vi "TCP Write.vi"(3 "error in (no error)":errorcluster, 4 "Data to Write":T1={"Array of Motor Speeds"=[0.0, 0.0, 0.0, 0.0]}, 5 "connection ID":refnum<k5>) -> (0 "error out":errorcluster, 2 "connection ID out":refnum<k5>)   [LabVIEW 2018]
uses:
  controls/TCP Write select.ctl
panel:
  # "Use this code as a starting point. This VI should take the values from the cluster\nand write them all on TCP."
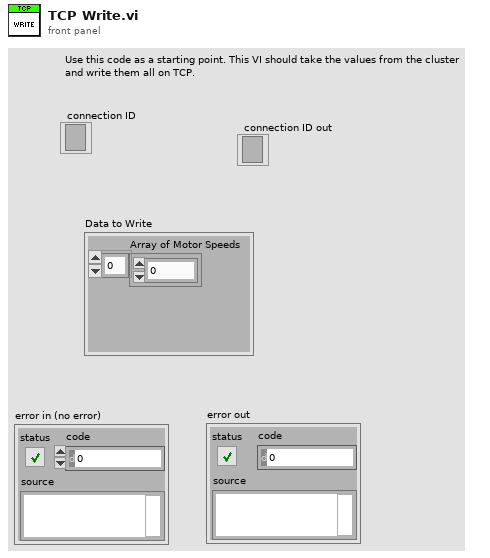
[diagram p1: front panel]
types:
  T1 = typedef "TCP Write select.ctl" = cluster{"Array of Motor Speeds":dbl[]}
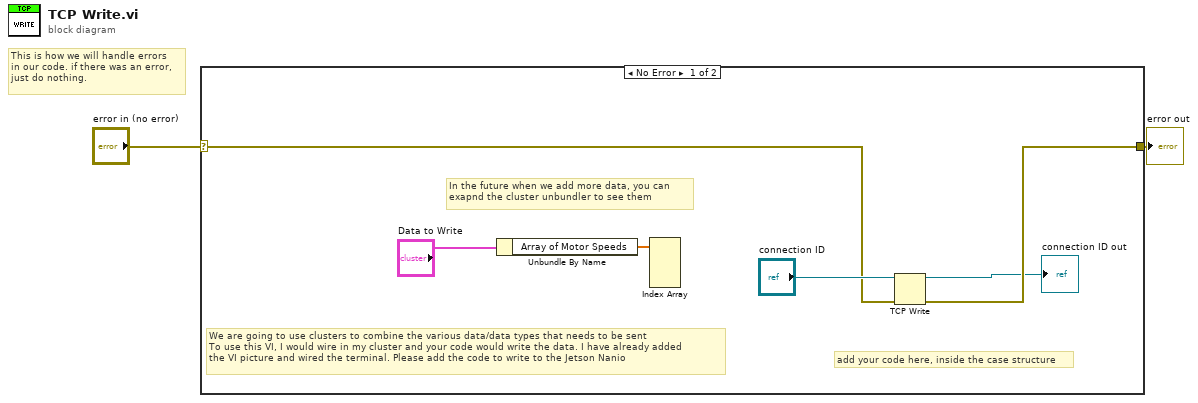
[diagram p0: block diagram]
diagram:
  # "This is how we will handle errors\nin our code. if there was an error,\njust do nothing."
  n1 = case shown="No Error" "error in (no error)" {
    selector: "error in (no error)" -> [w6 w9]
    tunnel: [w5 w9] -> w1
    frame No Error {
      # "add your code here, inside the case structure"
      # "In the future when we add more data, you can\nexapnd the cluster unbundler to see them"
      # "We are going to use clusters to combine the various data/data types that needs to be sent\nTo use this VI, I would wire in my cluster and your code would write the data. I have already added\nthe VI picture and wired the terminal. Please add the code to write to the Jetson Nanio"
      n2 = Unbundle By Name("Data to Write") -> ("Array of Motor Speeds"=w8:dbl[])
      n3 = Index Array(array=w8) -> ()  [unwired: 4 in, 4 out]
      n4 = TCP Write(connection ID="connection ID", error in (no error)=w6) -> (connection ID out=→"connection ID out":refnum<k5>, error out=w5:errorcluster)  [unwired: 2 in, 1 out]
    }
    frame Error {
      # "if there was an error, do nothing"
    }
  }
  "error out" <- w1
